vi "Set Force Cmd Bytes.vi"(10 "ForceCmdBytes":i32, 11 "DesktopModbus in":refnum<class "DesktopModbus.lvclass">) -> (3 "DesktopModbus out":refnum<class "DesktopModbus.lvclass">)   [LabVIEW 2016, in "DesktopModbus.lvclass"]
uses:
  DesktopModbus.lvclass
  DesktopModbus.lvclass/DesktopModbus.ctl
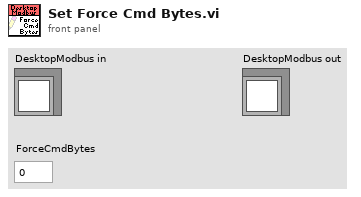
[diagram p1: front panel]
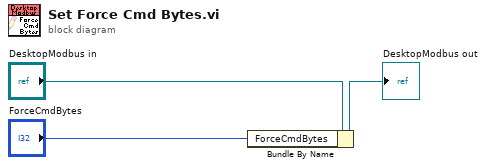
[diagram p0: block diagram]
diagram:
  n1 = Bundle By Name(cluster="DesktopModbus in", "ForceCmdBytes"="ForceCmdBytes") -> (→"DesktopModbus out":refnum<class "DesktopModbus.lvclass">)
